vi "CreatePrivateEvents.vi"(8 "error in (no error)":errorcluster, 11 "SMO.UI":refnum<class "SMO.UI.lvclass">) -> (0 "error out":errorcluster, 3 "SMO.UI out":refnum<class "SMO.UI.lvclass">)   [LabVIEW 2019, in "SMO.UI.lvclass"]
doc: "JKI State Machine Objects (SMO) 1.3.0.56\nJKI - JKI\nCopyright (c) 2017, JKI"
uses:
  SMO.UI.lvclass
  SMO.UI.lvclass/SMO.UI.ctl
  SMO/SMO.lvclass
panel:
  # "For instructions on how to use the JKI State Machine Objects, examples and video tutorials, visit:\nhttp://jki.net/state-machine-objects/\n\nJKI State Machine Objects™\nhttp://jki.net/state-machine-objects/\nCopyright (C) 2005-2015, JKI <info@jki.net>\nALL RIGHTS RESERVED"
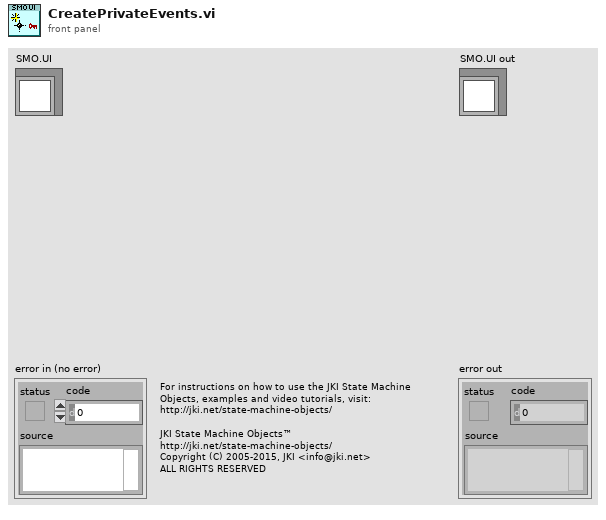
[diagram p1: front panel]
types:
  T1 = typedef "SMO.UI.lvclass/PrivateData--Ref.ctl" = refnum<data-value>
  T2 = typedef "SMO.UI.lvclass/PrivateData--Cluster.ctl" = cluster{"Public Events":T3, "Private Events":T4}
  T3 = typedef "SMO.UI.lvclass/PublicEvents--Cluster.ctl" = cluster{"UI Hidden":refnum<user-event>, "UI State":refnum<user-event>}
  T4 = typedef "SMO.UI.lvclass/PrivateEvents--Cluster.ctl" = cluster{"Show-Hide UI":refnum<user-event>}
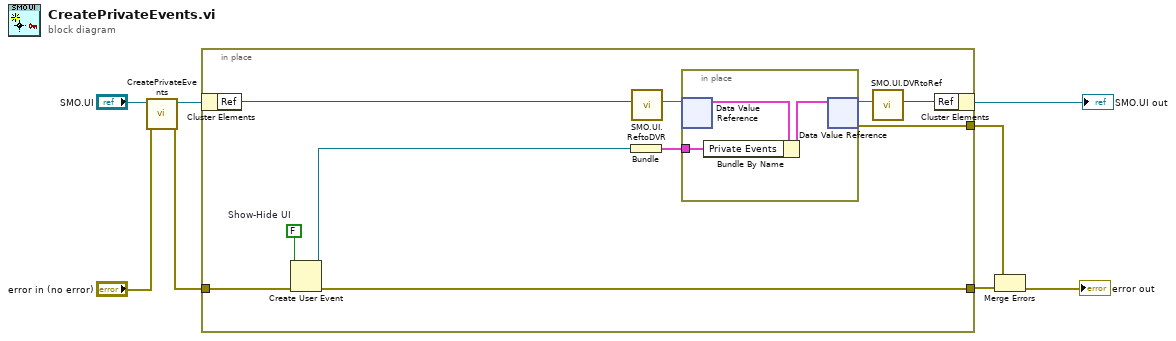
[diagram p0: block diagram]
diagram:
  n1 = call-parent "CreatePrivateEvents.vi"("error in (no error)"="error in (no error)", "SMO"="SMO.UI") -> ("error out"=w6:errorcluster, "SMO out"=w7:refnum<class "SMO.UI.lvclass">)  [unwired: 8 in]
  n2 = in-place {
    in-place-border: [w18] -> w3
    in-place-border: [w9] -> w4
    in-place-border: w6 -> [w10]
    w13 = FALSE  # Show-Hide UI
    n3 = in-place-cluster #1(w7) -> ("Ref"=w17:u32)
    n4 = Create User Event(user event datatype=w13, error in=w10) -> (user event=w11:refnum<user-event>, error out=w9:errorcluster)
    n5 = Bundle("Show-Hide UI"=w11) -> (w12:cluster{"Show-Hide UI":refnum<user-event>})  [unwired: 1 in]
    n6 = call "SMO.UI.ReftoDVR.vi"("Ref"=w17) -> ("Ref"=w16:T1)  [unwired: 10 in]
    n7 = in-place {
      in-place-border: w12 -> [w19]
      n8 = in-place-dvr #2(w16) -> (w21:T2)  [unwired: 1 out]
      n9 = Bundle By Name(cluster=w21, "Private Events"=w19) -> (w20:T2)
      n10 = in-place-dvr #2(w20) -> (w15:T1, w18:errorcluster)
    }
    n11 = call "SMO.UI.DVRtoRef.vi"("Ref"=w15) -> ("Ref"=w14:u32)  [unwired: 10 in]
    n12 = in-place-cluster #1("Ref"=w14) -> (→"SMO.UI out":refnum<class "SMO.UI.lvclass">)
  }
  n13 = Merge Errors(w3, w4) -> (→"error out":errorcluster)
